vi "实时小时数据单参数上传.vi"(0 "参数数值":T1={"CODMn"=TRUE, "CODCr"=TRUE, "DO"=TRUE, "铜"=TRUE, "PH"=TRUE, "氨氮"=TRUE, "比电导率"=TRUE, "水温"=TRUE, "盐度(海水)"=TRUE, "浊度"=TRUE, "总氮"=TRUE, "总磷"=TRUE, "叶绿素a"=TRUE, "藻密度"=TRUE, "水位"=TRUE, "流速"=TRUE, "瞬时流量"=TRUE, "累积流量"=TRUE}) -> (4 "数据发送起始时间":timestamp format="%<%.3X\n%Y/%m/%d>T", 6 "实时小时数据上传":bool, 15 "error out":errorcluster)   [LabVIEW 2016, in "数据传输系统.lvlib"]
uses:
  <vilib>/Utility/config.llb/Write Key (String).vi
  <vilib>/Utility/config.llb/NI_LVConfig.lvlib
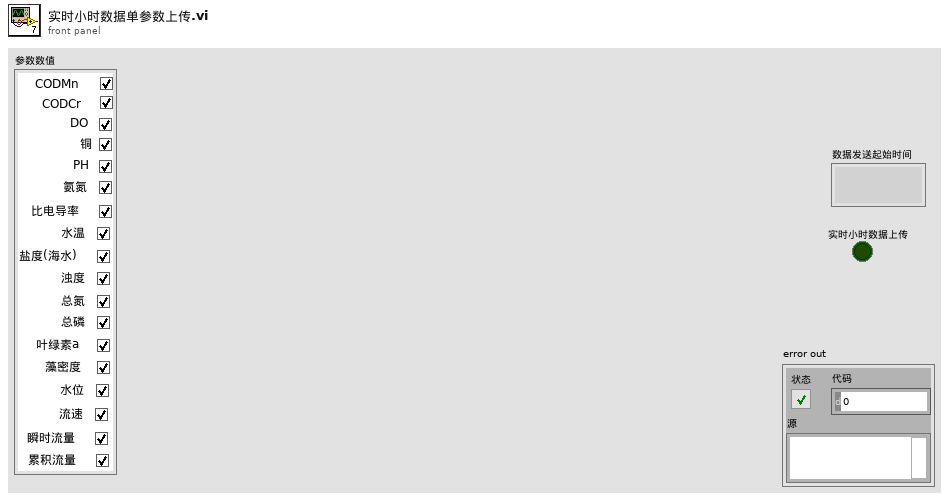
[diagram p1: front panel]
types:
  T1 = cluster{"CODMn":bool, "CODCr":bool, "DO":bool, "铜":bool, "PH":bool, "氨氮":bool, "比电导率":bool, "水温":bool, "盐度(海水)":bool, "浊度":bool, "总氮":bool, "总磷":bool, "叶绿素a":bool, "藻密度":bool, "水位":bool, "流速":bool, "瞬时流量":bool, "累积流量":bool}
  T2 = typedef "NI_LVConfig.lvlib/Config Data RefNum.ctl" = refnum<k1>
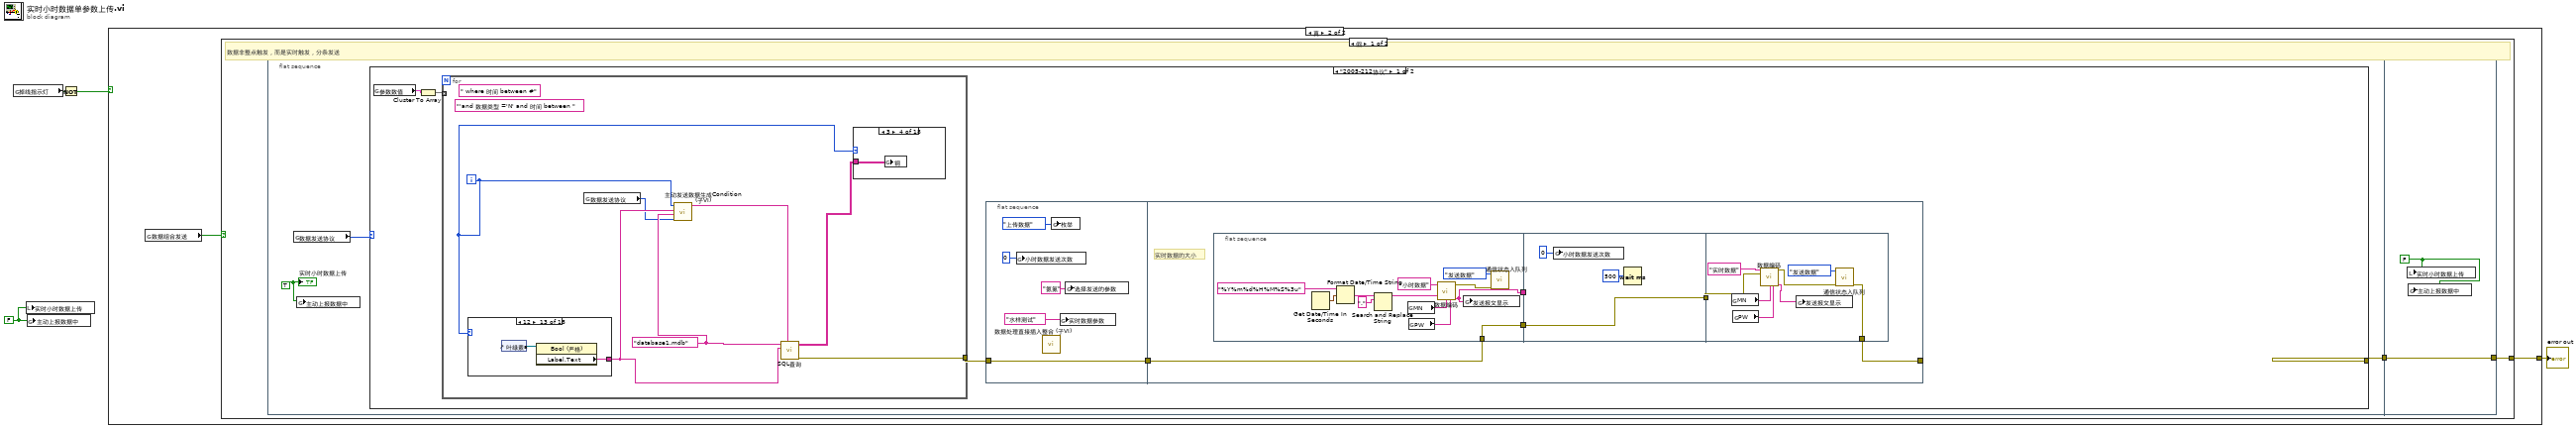
[diagram p0: block diagram]
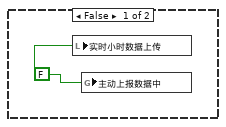
[diagram p2: hidden frame]
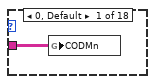
[diagram p3: hidden frame]
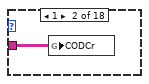
[diagram p4: hidden frame]
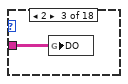
[diagram p5: hidden frame]
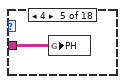
[diagram p6: hidden frame]
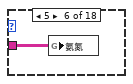
[diagram p7: hidden frame]
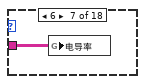
[diagram p8: hidden frame]
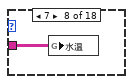
[diagram p9: hidden frame]
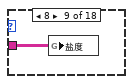
[diagram p10: hidden frame]
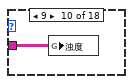
[diagram p11: hidden frame]
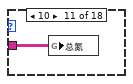
[diagram p12: hidden frame]
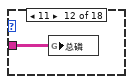
[diagram p13: hidden frame]
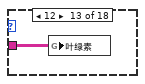
[diagram p14: hidden frame]
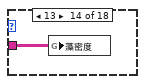
[diagram p15: hidden frame]
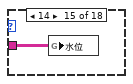
[diagram p16: hidden frame]
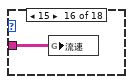
[diagram p17: hidden frame]
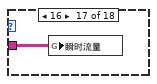
[diagram p18: hidden frame]
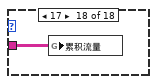
[diagram p19: hidden frame]
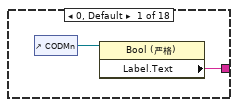
[diagram p20: hidden frame]
diagram:
  w4 = FALSE ("小时数据上传")
  n1 = global read "全局 数据发送重叠.vi" "掉线指示灯"() -> (w3:bool)
  n2 = local write "实时小时数据上传"(w4) -> ()
  n3 = global write "全局 数据发送重叠.vi" "主动上报数据中"(w4) -> ()
  n4 = Not(x=w3) -> (.not. x?=w2:bool)
  n5 = case shown="真" w2 {
    tunnel: [_ w7] -> w1
    frame False {
      w5 = FALSE ("小时数据上传")
      n6 = local write "实时小时数据上传"(w5) -> ()
      n7 = global write "全局 数据发送重叠.vi" "主动上报数据中"(w5) -> ()
    }
    frame True {
      n8 = global read "断电保存全局.vi" "数据组合发送"() -> (w6:bool)
      n9 = case shown="假" w6 {
        tunnel: [w8 _] -> w7
        frame False {
          # "数据非整点触发，而是实时触发，分条发送"
          n10 = flat-sequence {
            tunnel: [w12] -> w9
            tunnel: [w288] -> w8
            tunnel: w9 -> [w288]
            frame #0 {
              w11 = TRUE ("小时数据上传")
              n11 = global read "断电保存全局.vi" "数据发送协议"() -> (w10:enum16{"2005-212协议", "2017-212协议"})
              n12 = global write "全局 数据发送重叠.vi" "主动上报数据中"(w11) -> ()
              n13 = case shown="\"2005-212协议\"" w10 {
                tunnel: [_ w111] -> w12
                frame "2005-212协议" {
                  n14 = global read "全局1.vi" "参数数值"() -> (w13:T1)
                  n15 = Cluster To Array(cluster=w13) -> (array=w16:bool[])
                  n16 = for {
                    tunnel: w16 -> [_] mode=indexing
                    tunnel: [w56] -> w15
                    i -> [w54]
                    (unwired) " where 时间 between #"
                    w52 = "database1.mdb" ("database")
                    (unwired) "'and 数据类型 ='N' and 时间 between "
                    n17 = case shown="12" w54 {
                      tunnel: [w75 w77 w79 w81 w83 w85 w87 w89 w91 w93 w95 w97 w99 w101 w103 w105 w107 w109] -> w53
                      frame 0, Default {
                        n18 = control-ref of="CODMn"() -> (w76:refnum<vi>)
                        n19 = property class="Bool (严格)"(reference=w76) -> ("Label.Text"=w75:string)  [unwired: 1 in, 2 out]
                      }
                      frame 1 {
                        n20 = control-ref of="CODCr"() -> (w78:refnum<vi>)
                        n21 = property class="Bool (严格)"(reference=w78) -> ("Label.Text"=w77:string)  [unwired: 1 in, 2 out]
                      }
                      frame 2 {
                        n22 = control-ref of="DO"() -> (w80:refnum<vi>)
                        n23 = property class="Bool (严格)"(reference=w80) -> ("Label.Text"=w79:string)  [unwired: 1 in, 2 out]
                      }
                      frame 3 {
                        n24 = control-ref of="铜"() -> (w82:refnum<vi>)
                        n25 = property class="Bool (严格)"(reference=w82) -> ("Label.Text"=w81:string)  [unwired: 1 in, 2 out]
                      }
                      frame 4 {
                        n26 = control-ref of="PH"() -> (w84:refnum<vi>)
                        n27 = property class="Bool (严格)"(reference=w84) -> ("Label.Text"=w83:string)  [unwired: 1 in, 2 out]
                      }
                      frame 5 {
                        n28 = control-ref of="氨氮"() -> (w86:refnum<vi>)
                        n29 = property class="Bool (严格)"(reference=w86) -> ("Label.Text"=w85:string)  [unwired: 1 in, 2 out]
                      }
                      frame 6 {
                        n30 = control-ref of="比电导率"() -> (w88:refnum<vi>)
                        n31 = property class="Bool (严格)"(reference=w88) -> ("Label.Text"=w87:string)  [unwired: 1 in, 2 out]
                      }
                      frame 7 {
                        n32 = control-ref of="水温"() -> (w90:refnum<vi>)
                        n33 = property class="Bool (严格)"(reference=w90) -> ("Label.Text"=w89:string)  [unwired: 1 in, 2 out]
                      }
                      frame 8 {
                        n34 = control-ref of="盐度(海水)"() -> (w92:refnum<vi>)
                        n35 = property class="Bool (严格)"(reference=w92) -> ("Label.Text"=w91:string)  [unwired: 1 in, 2 out]
                      }
                      frame 9 {
                        n36 = control-ref of="浊度"() -> (w94:refnum<vi>)
                        n37 = property class="Bool (严格)"(reference=w94) -> ("Label.Text"=w93:string)  [unwired: 1 in, 2 out]
                      }
                      frame 10 {
                        n38 = control-ref of="总氮"() -> (w96:refnum<vi>)
                        n39 = property class="Bool (严格)"(reference=w96) -> ("Label.Text"=w95:string)  [unwired: 1 in, 2 out]
                      }
                      frame 11 {
                        n40 = control-ref of="总磷"() -> (w98:refnum<vi>)
                        n41 = property class="Bool (严格)"(reference=w98) -> ("Label.Text"=w97:string)  [unwired: 1 in, 2 out]
                      }
                      frame 12 {
                        n42 = control-ref of="叶绿素a"() -> (w100:refnum<vi>)
                        n43 = property class="Bool (严格)"(reference=w100) -> ("Label.Text"=w99:string)  [unwired: 1 in, 2 out]
                      }
                      frame 13 {
                        n44 = control-ref of="藻密度"() -> (w102:refnum<vi>)
                        n45 = property class="Bool (严格)"(reference=w102) -> ("Label.Text"=w101:string)  [unwired: 1 in, 2 out]
                      }
                      frame 14 {
                        n46 = control-ref of="水位"() -> (w104:refnum<vi>)
                        n47 = property class="Bool (严格)"(reference=w104) -> ("Label.Text"=w103:string)  [unwired: 1 in, 2 out]
                      }
                      frame 15 {
                        n48 = control-ref of="流速"() -> (w106:refnum<vi>)
                        n49 = property class="Bool (严格)"(reference=w106) -> ("Label.Text"=w105:string)  [unwired: 1 in, 2 out]
                      }
                      frame 16 {
                        n50 = control-ref of="瞬时流量"() -> (w108:refnum<vi>)
                        n51 = property class="Bool (严格)"(reference=w108) -> ("Label.Text"=w107:string)  [unwired: 1 in, 2 out]
                      }
                      frame 17 {
                        n52 = control-ref of="累积流量"() -> (w110:refnum<vi>)
                        n53 = property class="Bool (严格)"(reference=w110) -> ("Label.Text"=w109:string)  [unwired: 1 in, 2 out]
                      }
                    }
                    n54 = global read "断电保存全局.vi" "数据发送协议"() -> (w50:enum16{"2005-212协议", "2017-212协议"})
                    n55 = call "主动发送数据生成Condition(子VI).vi"("数据发送协议"=w50, "database"=w52, "Label.Text"=w53, "数值"=w54) -> ("CONDITION"=w51:string)  [unwired: 7 in]
                    n56 = call "SQL查询.vi"("condition"=w51, "table输入"=w53, "database"=w52) -> ("error out"=w56:errorcluster, "data"=w55:string[][])  [unwired: 7 in]
                    n57 = case shown="3" w54 {
                      tunnel: w55 -> [w57 w58 w59 w60 w61 w62 w63 w64 w65 w66 w67 w68 w69 w70 w71 w72 w73 w74]
                      frame 0, Default {
                        n58 = global write "全局 所有参数.vi" "CODMn"(w57) -> ()
                      }
                      frame 1 {
                        n59 = global write "全局 所有参数.vi" "CODCr"(w58) -> ()
                      }
                      frame 2 {
                        n60 = global write "全局 所有参数.vi" "DO"(w59) -> ()
                      }
                      frame 3 {
                        n61 = global write "全局 所有参数.vi" "铜"(w60) -> ()
                      }
                      frame 4 {
                        n62 = global write "全局 所有参数.vi" "PH"(w61) -> ()
                      }
                      frame 5 {
                        n63 = global write "全局 所有参数.vi" "氨氮"(w62) -> ()
                      }
                      frame 6 {
                        n64 = global write "全局 所有参数.vi" "电导率"(w63) -> ()
                      }
                      frame 7 {
                        n65 = global write "全局 所有参数.vi" "水温"(w64) -> ()
                      }
                      frame 8 {
                        n66 = global write "全局 所有参数.vi" "盐度"(w65) -> ()
                      }
                      frame 9 {
                        n67 = global write "全局 所有参数.vi" "浊度"(w66) -> ()
                      }
                      frame 10 {
                        n68 = global write "全局 所有参数.vi" "总氮"(w67) -> ()
                      }
                      frame 11 {
                        n69 = global write "全局 所有参数.vi" "总磷"(w68) -> ()
                      }
                      frame 12 {
                        n70 = global write "全局 所有参数.vi" "叶绿素"(w69) -> ()
                      }
                      frame 13 {
                        n71 = global write "全局 所有参数.vi" "藻密度"(w70) -> ()
                      }
                      frame 14 {
                        n72 = global write "全局 所有参数.vi" "水位"(w71) -> ()
                      }
                      frame 15 {
                        n73 = global write "全局 所有参数.vi" "流速"(w72) -> ()
                      }
                      frame 16 {
                        n74 = global write "全局 所有参数.vi" "瞬时流量"(w73) -> ()
                      }
                      frame 17 {
                        n75 = global write "全局 所有参数.vi" "累积流量"(w74) -> ()
                      }
                    }
                  }
                  n76 = flat-sequence {
                    tunnel: w15 -> [w17]
                    tunnel: [w17] -> w14
                    tunnel: w14 -> [w23]
                    tunnel: [w22] -> _
                    frame #0 {
                      n77 = global write "全局 小时数据发送次数.vi" "小时数据发送次数"(0 ("小时数据发送次数")) -> ()
                      n78 = call "数据处理直接插入整合 (子VI).vi"() -> ()  [unwired: 12 in]
                      n79 = global write "全局1.vi" "枚举"(enum16{"返回请求应答", "上传数据", "返回执行结果"}."上传数据" ("枚举")) -> ()
                      n80 = global write "全局 实时数据参数.vi" "实时数据参数"("水样测试" ("实时数据参数")) -> ()
                      n81 = global write "全局 水样时间.vi" "选择发送的参数"("氨氮" ("选择发送的参数")) -> ()
                    }
                    frame #1 {
                      # "实时数据的大小"
                      n82 = flat-sequence {
                        tunnel: [w32] -> w26
                        tunnel: [w27] -> w24
                        tunnel: w23 -> [w27]
                        tunnel: w26 -> [_]
                        tunnel: [w40] -> w25
                        tunnel: w24 -> [w40]
                        tunnel: w25 -> [w48]
                        tunnel: [w42] -> w22
                        frame #0 {
                          n83 = Get Date/Time In Seconds() -> (seconds since 1Jan1904=w35:timestamp)
                          n84 = Format Date/Time String(time format string (%c)="%Y%m%d%H%M%S%3u" ("时间格式字符串(%c)"), seconds (now)=w35) -> (date/time string=w36:string)  [unwired: 1 in]
                          n85 = Search and Replace String(input string=w36, search string="." ("搜索字符串")) -> (result string=w38:string)  [unwired: 6 in, 3 out]
                          n86 = global read "断电保存全局.vi" "MN"() -> (w30:string)
                          n87 = global read "断电保存全局.vi" "PW"() -> (w29:string)
                          n88 = call "数据编码.vi"("table输入"="小时数据" ("新元素/子数组"), "QN"=w38, "MN"=w30, "PW"=w29) -> ("错误常量"=w28:errorcluster, "通讯包字符串"=w32:string)  [unwired: 10 in]
                          n89 = global write "全局1.vi" "发送报文显示"(w32) -> ()
                          n90 = call "通信状态入队列.vi"("错误输入（无错误）"=w28, "枚举"=enum16{"打开连接", "发送数据", "读取数据", "数据处理", "关闭连接"}."发送数据") -> ()  [unwired: 9 in, 1 out]
                        }
                        frame #1 {
                          n91 = global write "全局 小时数据发送次数.vi" "小时数据发送次数"(0 ("小时数据发送次数")) -> ()
                          n92 = Wait (ms)(milliseconds to wait=u32 500 ("等待时间（毫秒）")) -> ()  [unwired: 1 out]
                        }
                        frame #2 {
                          n93 = global read "断电保存全局.vi" "MN"() -> (w44:string)
                          n94 = global read "断电保存全局.vi" "PW"() -> (w45:string)
                          n95 = call "数据编码.vi"("table输入"="实时数据" ("新元素/子数组"), "错误常量 2"=w48, "MN"=w44, "PW"=w45) -> ("错误常量"=w43:errorcluster, "通讯包字符串"=w47:string)  [unwired: 10 in]
                          n96 = global write "全局1.vi" "发送报文显示"(w47) -> ()
                          n97 = call "通信状态入队列.vi"("错误输入（无错误）"=w43, "枚举"=enum16{"打开连接", "发送数据", "读取数据", "数据处理", "关闭连接"}."发送数据") -> ("错误输出"=w42:errorcluster)  [unwired: 9 in]
                        }
                      }
                    }
                  }
                }
                frame "2017-212协议", Default {
                  n98 = local read "参数数值"() -> (w113:T1)
                  n99 = Cluster To Array(cluster=w113) -> (array=w112:bool[])
                  n100 = for {
                    tunnel: w112 -> [_] mode=indexing
                    tunnel: [w118] -> w111
                    tunnel: [w118] -> _
                    i -> [w117]
                    (unwired) " where 时间 between #"
                    w116 = "database1.mdb" ("database")
                    (unwired) "'and 数据类型 ='N' and 时间 between "
                    w132 = 0 ("索引 (行)")
                    n101 = case shown="3" w117 {
                      tunnel: [w251 w253 w255 w257 w259 w261 w263 w265 w267 w269 w271 w273 w275 w277 w279 w281 w283 w285] -> w115
                      frame 0, Default {
                        n102 = control-ref of="CODMn"() -> (w252:refnum<vi>)
                        n103 = property class="Bool (严格)"(reference=w252) -> ("Label.Text"=w251:string)  [unwired: 1 in, 2 out]
                      }
                      frame 1 {
                        n104 = control-ref of="CODCr"() -> (w254:refnum<vi>)
                        n105 = property class="Bool (严格)"(reference=w254) -> ("Label.Text"=w253:string)  [unwired: 1 in, 2 out]
                      }
                      frame 2 {
                        n106 = control-ref of="DO"() -> (w256:refnum<vi>)
                        n107 = property class="Bool (严格)"(reference=w256) -> ("Label.Text"=w255:string)  [unwired: 1 in, 2 out]
                      }
                      frame 3 {
                        n108 = control-ref of="铜"() -> (w258:refnum<vi>)
                        n109 = property class="Bool (严格)"(reference=w258) -> ("Label.Text"=w257:string)  [unwired: 1 in, 2 out]
                      }
                      frame 4 {
                        n110 = control-ref of="PH"() -> (w260:refnum<vi>)
                        n111 = property class="Bool (严格)"(reference=w260) -> ("Label.Text"=w259:string)  [unwired: 1 in, 2 out]
                      }
                      frame 5 {
                        n112 = control-ref of="氨氮"() -> (w262:refnum<vi>)
                        n113 = property class="Bool (严格)"(reference=w262) -> ("Label.Text"=w261:string)  [unwired: 1 in, 2 out]
                      }
                      frame 6 {
                        n114 = control-ref of="比电导率"() -> (w264:refnum<vi>)
                        n115 = property class="Bool (严格)"(reference=w264) -> ("Label.Text"=w263:string)  [unwired: 1 in, 2 out]
                      }
                      frame 7 {
                        n116 = control-ref of="水温"() -> (w266:refnum<vi>)
                        n117 = property class="Bool (严格)"(reference=w266) -> ("Label.Text"=w265:string)  [unwired: 1 in, 2 out]
                      }
                      frame 8 {
                        n118 = control-ref of="盐度(海水)"() -> (w268:refnum<vi>)
                        n119 = property class="Bool (严格)"(reference=w268) -> ("Label.Text"=w267:string)  [unwired: 1 in, 2 out]
                      }
                      frame 9 {
                        n120 = control-ref of="浊度"() -> (w270:refnum<vi>)
                        n121 = property class="Bool (严格)"(reference=w270) -> ("Label.Text"=w269:string)  [unwired: 1 in, 2 out]
                      }
                      frame 10 {
                        n122 = control-ref of="总氮"() -> (w272:refnum<vi>)
                        n123 = property class="Bool (严格)"(reference=w272) -> ("Label.Text"=w271:string)  [unwired: 1 in, 2 out]
                      }
                      frame 11 {
                        n124 = control-ref of="总磷"() -> (w274:refnum<vi>)
                        n125 = property class="Bool (严格)"(reference=w274) -> ("Label.Text"=w273:string)  [unwired: 1 in, 2 out]
                      }
                      frame 12 {
                        n126 = control-ref of="叶绿素a"() -> (w276:refnum<vi>)
                        n127 = property class="Bool (严格)"(reference=w276) -> ("Label.Text"=w275:string)  [unwired: 1 in, 2 out]
                      }
                      frame 13 {
                        n128 = control-ref of="藻密度"() -> (w278:refnum<vi>)
                        n129 = property class="Bool (严格)"(reference=w278) -> ("Label.Text"=w277:string)  [unwired: 1 in, 2 out]
                      }
                      frame 14 {
                        n130 = control-ref of="水位"() -> (w280:refnum<vi>)
                        n131 = property class="Bool (严格)"(reference=w280) -> ("Label.Text"=w279:string)  [unwired: 1 in, 2 out]
                      }
                      frame 15 {
                        n132 = control-ref of="流速"() -> (w282:refnum<vi>)
                        n133 = property class="Bool (严格)"(reference=w282) -> ("Label.Text"=w281:string)  [unwired: 1 in, 2 out]
                      }
                      frame 16 {
                        n134 = control-ref of="瞬时流量"() -> (w284:refnum<vi>)
                        n135 = property class="Bool (严格)"(reference=w284) -> ("Label.Text"=w283:string)  [unwired: 1 in, 2 out]
                      }
                      frame 17 {
                        n136 = control-ref of="累积流量"() -> (w286:refnum<vi>)
                        n137 = property class="Bool (严格)"(reference=w286) -> ("Label.Text"=w285:string)  [unwired: 1 in, 2 out]
                      }
                    }
                    n138 = global read "断电保存全局.vi" "数据发送协议"() -> (w114:enum16{"2005-212协议", "2017-212协议"})
                    n139 = call "主动发送数据生成Condition(子VI).vi"("数据发送协议"=w114, "database"=w116, "Label.Text"=w115, "数值"=w117) -> ("CONDITION"=w134:string)  [unwired: 7 in]
                    n140 = call "SQL查询.vi"("condition"=w134, "table输入"=w115, "database"=w116) -> ("error out"=w118:errorcluster, "data"=w130:string[][])  [unwired: 7 in]
                    n141 = Empty Array?(array=w130) -> (empty?=w133:bool)
                    n142 = call "短日期时间转长日期格式.vi"("data"=w130) -> ("输出数组"=w131:string[][])  [unwired: 10 in]
                    n143 = Not(x=w133) -> (.not. x?=w127:bool)
                    n144 = Index Array(array=w131, index (row)=w132, index (col)=w132) -> (element=w124:string)
                    n145 = global write "全局 水样时间.vi" "选择发送的参数"(w115) -> ()
                    n146 = flat-sequence {
                      tunnel: [w142] -> w129
                      tunnel: [w141] -> w128
                      tunnel: w127 -> [w142]
                      tunnel: w130 -> [w141]
                      tunnel: w117 -> [w136]
                      tunnel: w115 -> [w138]
                      tunnel: [w138] -> w125
                      tunnel: w124 -> [w137]
                      tunnel: [w137] -> w122
                      tunnel: [w136] -> w119
                      tunnel: w129 -> [w162]
                      tunnel: w128 -> [w165]
                      tunnel: [w164] -> w126
                      tunnel: w125 -> [w164]
                      tunnel: [w163] -> w123
                      tunnel: w122 -> [w163]
                      tunnel: [w162] -> w121
                      tunnel: [w161] -> w120
                      tunnel: w119 -> [w161]
                      tunnel: w126 -> [w219]
                      tunnel: w123 -> [w218]
                      tunnel: w121 -> [w216]
                      tunnel: w120 -> [w217]
                      frame #0 {
                        n147 = case shown="3" w136 {
                          tunnel: w141 -> [w143 w144 w145 w146 w147 w148 w149 w150 w151 w152 w153 w154 w155 w156 w157 w158 w159 w160]
                          frame 0, Default {
                            n148 = global write "全局 所有参数.vi" "CODMn"(w143) -> ()
                          }
                          frame 1 {
                            n149 = global write "全局 所有参数.vi" "CODCr"(w144) -> ()
                          }
                          frame 2 {
                            n150 = global write "全局 所有参数.vi" "DO"(w145) -> ()
                          }
                          frame 3 {
                            n151 = global write "全局 所有参数.vi" "铜"(w146) -> ()
                          }
                          frame 4 {
                            n152 = global write "全局 所有参数.vi" "PH"(w147) -> ()
                          }
                          frame 5 {
                            n153 = global write "全局 所有参数.vi" "氨氮"(w148) -> ()
                          }
                          frame 6 {
                            n154 = global write "全局 所有参数.vi" "电导率"(w149) -> ()
                          }
                          frame 7 {
                            n155 = global write "全局 所有参数.vi" "水温"(w150) -> ()
                          }
                          frame 8 {
                            n156 = global write "全局 所有参数.vi" "盐度"(w151) -> ()
                          }
                          frame 9 {
                            n157 = global write "全局 所有参数.vi" "浊度"(w152) -> ()
                          }
                          frame 10 {
                            n158 = global write "全局 所有参数.vi" "总氮"(w153) -> ()
                          }
                          frame 11 {
                            n159 = global write "全局 所有参数.vi" "总磷"(w154) -> ()
                          }
                          frame 12 {
                            n160 = global write "全局 所有参数.vi" "叶绿素"(w155) -> ()
                          }
                          frame 13 {
                            n161 = global write "全局 所有参数.vi" "藻密度"(w156) -> ()
                          }
                          frame 14 {
                            n162 = global write "全局 所有参数.vi" "水位"(w157) -> ()
                          }
                          frame 15 {
                            n163 = global write "全局 所有参数.vi" "流速"(w158) -> ()
                          }
                          frame 16 {
                            n164 = global write "全局 所有参数.vi" "瞬时流量"(w159) -> ()
                          }
                          frame 17 {
                            n165 = global write "全局 所有参数.vi" "累积流量"(w160) -> ()
                          }
                        }
                        n166 = global write "全局 小时数据发送次数.vi" "小时数据发送次数"(0 ("小时数据发送次数")) -> ()
                        n167 = global write "全局 数据发送重叠.vi" "数据接收超时指示灯"(FALSE ("数据接收超时指示灯")) -> ()
                        n168 = global write "全局1.vi" "枚举"(enum16{"返回请求应答", "上传数据", "返回执行结果"}."上传数据" ("枚举")) -> ()
                      }
                      frame #1 {
                        n169 = case shown="真" w162 {
                          tunnel: w165 -> [_ w168]
                          tunnel: w161 -> [_ w167]
                          tunnel: w161 -> [_ w166]
                          frame False {
                          }
                          frame True {
                            n170 = for {
                              tunnel: w168 -> [_] mode=indexing
                              tunnel: w167 -> [w185]
                              tunnel: w166 -> [w184]
                              # "实时数据的大小"
                              n171 = Wait (ms)(milliseconds to wait=u32 500 ("等待时间（毫秒）")) -> ()  [unwired: 1 out]
                              n172 = global write "全局 实时数据参数.vi" "实时数据参数"("水样测试" ("实时数据参数")) -> ()
                              n173 = Get Date/Time In Seconds() -> (seconds since 1Jan1904=w179:timestamp)
                              n174 = Format Date/Time String(time format string (%c)="%Y%m%d%H%M%S%3u" ("时间格式字符串(%c)"), seconds (now)=w179) -> (date/time string=w180:string)  [unwired: 1 in]
                              n175 = Search and Replace String(input string=w180, search string="." ("搜索字符串")) -> (result string=w182:string)  [unwired: 6 in, 3 out]
                              n176 = global read "断电保存全局.vi" "MN"() -> (w175:string)
                              n177 = global read "断电保存全局.vi" "PW"() -> (w174:string)
                              n178 = global read "断电保存全局.vi" "判断数据反馈"() -> (w171:bool)
                              n179 = call "数据编码.vi"("table输入"="小时数据" ("新元素/子数组"), "QN"=w182, "MN"=w175, "PW"=w174) -> ("错误常量"=w172:errorcluster, "通讯包字符串"=w169:string)  [unwired: 10 in]
                              n180 = global write "全局1.vi" "发送报文显示"(w169) -> ()
                              n181 = call "通信状态入队列.vi"("错误输入（无错误）"=w172, "枚举"=enum16{"打开连接", "发送数据", "读取数据", "数据处理", "关闭连接"}."发送数据") -> ()  [unwired: 9 in, 1 out]
                              n182 = case shown="真" w171 {
                                tunnel: [_ w206] -> w183
                                tunnel: w169 -> [_ w205]
                                tunnel: w185 -> [_ w204]
                                frame False {
                                }
                                frame True {
                                n183 = case shown="0, 默认" w204 {
                                tunnel: [w208 _] -> w206
                                tunnel: w205 -> [w207 _]
                                frame 0, Default {
                                n184 = Empty String/Path?(string/path=w207) -> (empty?=w209:bool)
                                n185 = case shown="假" w209 {
                                tunnel: [w212 _] -> w208
                                tunnel: w207 -> [w211 _]
                                frame False {
                                n186 = global read "断电保存全局.vi" "数据发送通道"() -> (w210:enum16{"TCP", "VISA"})
                                n187 = call "数据补发判定有限循环.vi"("数据输入"=w211, "数据发送通道"=w210) -> ("error out"=w212:errorcluster)  [unwired: 9 in]
                                }
                                frame True {
                                }
                                }
                                }
                                frame 14..17 {
                                }
                                }
                                }
                              }
                              n188 = global read "断电保存全局.vi" "2011发送"() -> (w170:bool)
                              n189 = case shown="真" w170 {
                                tunnel: w184 -> [_ w197]
                                tunnel: w183 -> [_ w196]
                                frame False {
                                }
                                frame True {
                                n190 = global read "断电保存全局.vi" "MN"() -> (w191:string)
                                n191 = global read "断电保存全局.vi" "PW"() -> (w190:string)
                                n192 = global write "全局 实时数据参数.vi" "实时数据参数"("水样测试" ("实时数据参数")) -> ()
                                n193 = call "数据编码.vi"("table输入"="实时数据" ("新元素/子数组"), "错误常量 2"=w196, "MN"=w191, "PW"=w190) -> ("错误常量"=w192:errorcluster, "通讯包字符串"=w187:string)  [unwired: 10 in]
                                n194 = global write "全局1.vi" "发送报文显示"(w187) -> ()
                                n195 = call "通信状态入队列.vi"("错误输入（无错误）"=w192, "枚举"=enum16{"打开连接", "发送数据", "读取数据", "数据处理", "关闭连接"}."发送数据") -> ("错误输出"=w189:errorcluster)  [unwired: 9 in]
                                n196 = global read "断电保存全局.vi" "判断数据反馈"() -> (w188:bool)
                                n197 = case shown="真" w188 {
                                tunnel: w187 -> [_ w200]
                                tunnel: w189 -> [_ w199]
                                tunnel: w197 -> [_ w198]
                                frame False {
                                }
                                frame True {
                                n198 = case shown="0, 默认" w198 {
                                tunnel: w200 -> [w203 _]
                                tunnel: w199 -> [w202 _]
                                frame 0, Default {
                                n199 = global read "断电保存全局.vi" "数据发送通道"() -> (w201:enum16{"TCP", "VISA"})
                                n200 = call "数据补发判定有限循环.vi"("错误输入（无错误）"=w202, "数据输入"=w203, "数据发送通道"=w201) -> ()  [unwired: 8 in, 1 out]
                                }
                                frame 14..17 {
                                }
                                }
                                }
                                }
                                }
                              }
                            }
                          }
                        }
                      }
                      frame #2 {
                        n201 = global read "全局 数据发送重叠.vi" "数据接收超时指示灯"() -> (w213:bool)
                        n202 = Not(x=w213) -> (.not. x?=w214:bool)
                        n203 = Compound Arithmetic op=AND ("复合运算")(w214, w216) -> (w215:bool)
                        n204 = case shown="真" w215 {
                          tunnel: w218 -> [_ w222]
                          tunnel: w217 -> [_ w232]
                          tunnel: w219 -> [_ w223]
                          frame False {
                          }
                          frame True {
                            n205 = call "日期时间字符串转换分钟数加一.vi"("data[0]"=w222) -> ("日期/时间字符串"=w221:string)  [unwired: 10 in]
                            n206 = call "时间日期字符串至时间标识转换.vi"("时间日期字符串"=w221) -> ("时间标识"=→"数据发送起始时间":timestamp)  [unwired: 10 in]
                            n207 = call <vilib>:"Application Directory.vi"() -> ("Application Directory"=w224:path)
                            n208 = case shown="3" w232 {
                              tunnel: w221 -> [w233 w234 w235 w236 w237 w238 w239 w240 w241 w242 w243 w244 w245 w246 w247 w248 w249 w250]
                              frame 0, Default {
                                n209 = global write "全局 水样时间.vi" "time1"(w233) -> ()
                              }
                              frame 1 {
                                n210 = global write "全局 水样时间.vi" "time2"(w234) -> ()
                              }
                              frame 2 {
                                n211 = global write "全局 水样时间.vi" "time3"(w235) -> ()
                              }
                              frame 3 {
                                n212 = global write "全局 水样时间.vi" "time4"(w236) -> ()
                              }
                              frame 4 {
                                n213 = global write "全局 水样时间.vi" "time5"(w237) -> ()
                              }
                              frame 5 {
                                n214 = global write "全局 水样时间.vi" "time6"(w238) -> ()
                              }
                              frame 6 {
                                n215 = global write "全局 水样时间.vi" "time7"(w239) -> ()
                              }
                              frame 7 {
                                n216 = global write "全局 水样时间.vi" "time8"(w240) -> ()
                              }
                              frame 8 {
                                n217 = global write "全局 水样时间.vi" "time9"(w241) -> ()
                              }
                              frame 9 {
                                n218 = global write "全局 水样时间.vi" "time10"(w242) -> ()
                              }
                              frame 10 {
                                n219 = global write "全局 水样时间.vi" "time11"(w243) -> ()
                              }
                              frame 11 {
                                n220 = global write "全局 水样时间.vi" "time12"(w244) -> ()
                              }
                              frame 12 {
                                n221 = global write "全局 水样时间.vi" "time13"(w245) -> ()
                              }
                              frame 13 {
                                n222 = global write "全局 水样时间.vi" "time14"(w246) -> ()
                              }
                              frame 14 {
                                n223 = global write "全局 水样时间.vi" "time15"(w247) -> ()
                              }
                              frame 15 {
                                n224 = global write "全局 水样时间.vi" "time16"(w248) -> ()
                              }
                              frame 16 {
                                n225 = global write "全局 水样时间.vi" "time17"(w249) -> ()
                              }
                              frame 17 {
                                n226 = global write "全局 水样时间.vi" "time18"(w250) -> ()
                              }
                            }
                            n227 = Build Path(base path=w224, name or relative path="data\\Set.ini" ("名称或相对路径")) -> (appended path=w226:path)
                            n228 = call <vilib>:"Open Config Data.vi"("configuration file path"=w226) -> ("error out"=w228:errorcluster, "refnum"=w227:T2)  [unwired: 8 in, 1 out]
                            n229 = call-poly <vilib>:"Write Key.vi"("section"="线程一数据搜索起始时间", "error in (no error)"=w228, "value"=w221, "key"=w223, "refnum"=w227) -> ("error out"=w230:errorcluster, "refnum out"=w229:T2)  [unwired: 4 in, 1 out]
                            n230 = call <vilib>:"Close Config Data.vi"("error in (no error)"=w230, "refnum"=w229) -> ()  [unwired: 8 in, 2 out]
                          }
                        }
                      }
                    }
                  }
                }
              }
              "实时小时数据上传" <- w11
            }
            frame #1 {
              w287 = FALSE ("小时数据上传")
              n231 = local write "实时小时数据上传"(w287) -> ()
              n232 = global write "全局 数据发送重叠.vi" "主动上报数据中"(w287) -> ()
            }
          }
        }
        frame True {
          # "数据整点触发，整条发送"
        }
      }
    }
  }
  "error out" <- w1
